vi "voltagetopressure.vi"(1 "Input":dbl(slide) scale=0.0..10.0) -> (0 "Output":dbl)   [LabVIEW 2011]
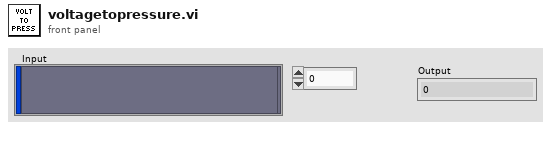
[diagram p1: front panel]
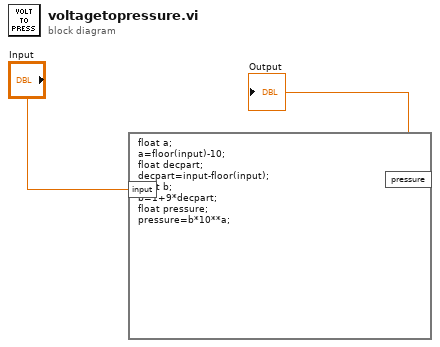
[diagram p0: block diagram]
diagram:
  n1 = formula code="float a;\na=floor(input)-10;\nfloat decpart;\ndecpart=input-floor(input);\nfloat b;\nb=1+9*decpart;\nfloat pressure;\npressure=b*10**a;"("input"="Input") -> ("pressure"=→"Output":dbl)
